vi "DataLog Subsets Actor.vi"(0 "action":T1, 5 "tag":string, 7 "subsets in":T2[](array[typedef]), 9 "tag config list":T3[](array[typedef]) {"logging parameters" format="%.2e"; "precision" items=["0", "1", "2", "3", "4", "5", "6", "7", "8", "9", "10", "11", "12", "13", "14", "15", "16", "17"]; "limit delay" format="%.2e"; "deadband" format="%.2e"}, 11 "error in (no error)":errorcluster, 12 "database path":path, 13 "new name":string) -> (4 "changes":bool, 8 "subset out":T2[](array[typedef]), 15 "error out":errorcluster)   [LabVIEW 2012]
doc: "Implements several actions designed to keep the in-memory and on-disk lists of tag subsets in sync with modifications to the tags list of their database."
uses:
  typedefs/t_Datalog Subsets Actions.ctl
  typedefs/clusters/t_DataLog Tag Subset.ctl
  typedefs/clusters/t_DataLog Tag Config.ctl
  typedefs/t_DataLog Temporal Types.ctl
  typedefs/t_DataLog Value Types.ctl
  typedefs/t_DataLog Numerical Format.ctl
  typedefs/t_DataLog Logging Algorithms.ctl
  glb_DataLog MCVD.vi
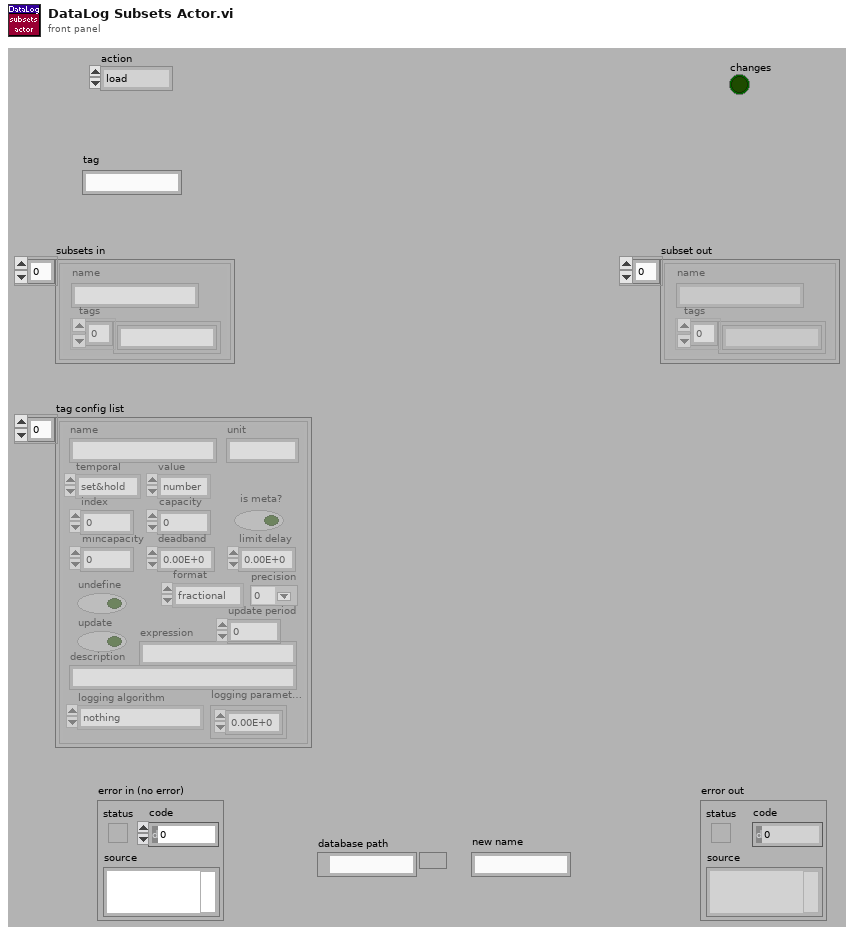
[diagram p1: front panel]
types:
  T1 = typedef "t_Datalog Subsets Actions.ctl" = enum16{"load", "rename", "delete", "save"}
  T2 = typedef "t_DataLog Tag Subset.ctl" = cluster{"name":string, "tags":string[]}
  T3 = typedef "t_DataLog Tag Config.ctl" = cluster{"name":string, "unit":string, "temporal":T4, "value":T5, "index":i32, "capacity":i32, "is meta?":bool, "mincapacity":i32, "deadband":dbl, "limit delay":dbl, "format":T6, "precision":u8, "undefine":bool, "update":bool, "update period":u16, "expression":string, "description":string, "logging algorithm":T7, "logging parameters":dbl[]}
  T4 = typedef "t_DataLog Temporal Types.ctl" = enum16{"set&hold", "sample", "event"}
  T5 = typedef "t_DataLog Value Types.ctl" = enum16{"number", "string"}
  T6 = typedef "t_DataLog Numerical Format.ctl" = enum8{"fractional", "exponential", "engineering"}
  T7 = typedef "t_DataLog Logging Algorithms.ctl" = enum16{"nothing", "changes", "everything", "every Nth", "time threshold", "value threshold + prior", "t or v threshold", "t or v threshold + prior"}
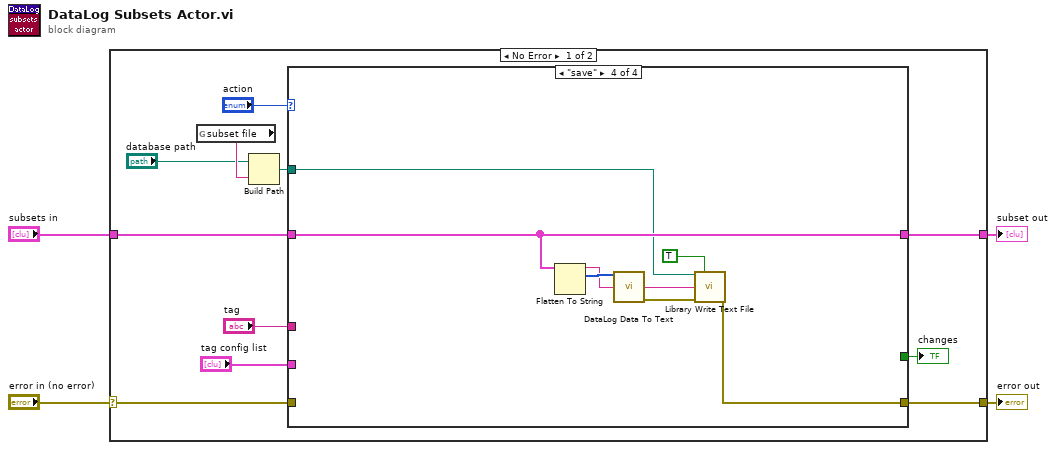
[diagram p0: block diagram]
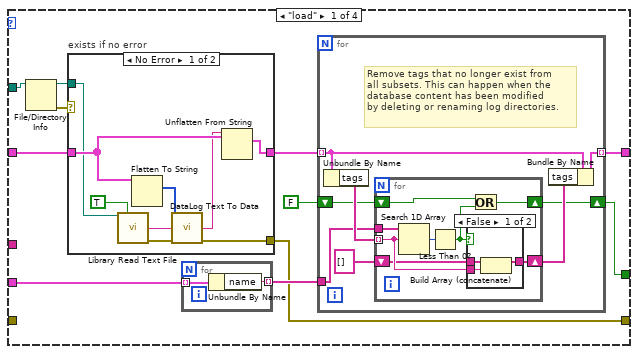
[diagram p2: hidden frame]
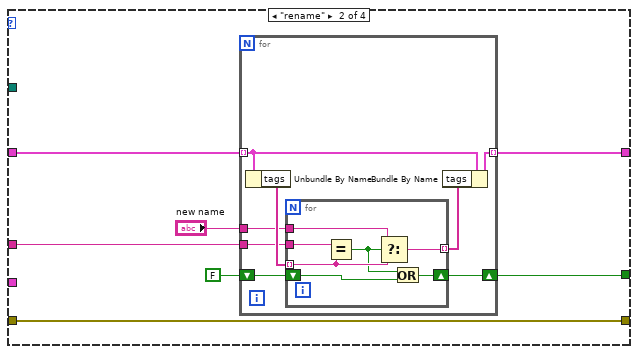
[diagram p5: hidden frame]
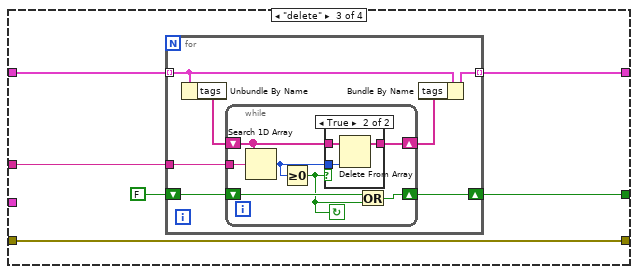
[diagram p6: hidden frame]
diagram:
  n1 = case shown="No Error" "error in (no error)" {
    selector: "error in (no error)" -> [w12 w112]
    tunnel: [w15 w113] -> w4
    tunnel: "subsets in" -> [w14 w113]
    tunnel: [w13 w112] -> w1
    frame No Error {
      n2 = global read "glb_DataLog MCVD.vi" "subset file"() -> (w8:string)
      n3 = Build Path(base path="database path", name or relative path=w8) -> (appended path=w6:path)
      n4 = case shown="\"save\"" "action" {
        tunnel: [w25 w64 w80 w105] -> w15
        tunnel: w14 -> [w23 w63 w85 w105]
        tunnel: [w20 w62 w84 w106] -> w13
        tunnel: w12 -> [_ w62 w84 _]
        tunnel: "tag" -> [_ w61 w83 _]
        tunnel: "tag config list" -> [w19 _ _ _]
        tunnel: w6 -> [w18 _ _ w104]
        tunnel: [w16 w59 w81 _] -> w5
        frame "load" {
          n5 = File/Directory Info(path=w18) -> (path out=w22:path, error out=w21:errorcluster)  [unwired: 1 in, 5 out]
          n6 = case "exists if no error" shown="No Error" w21 {
            tunnel: w23 -> [w53 _]
            tunnel: [w54 _] -> w24
            tunnel: [w51 _] -> w20
            tunnel: w22 -> [w50 _]
            frame No Error {
              n7 = call "Library Read Text File.vi"("file path"=w50, "convert eol (F)"=TRUE) -> ("read text"=w57:string, "error out"=w56:errorcluster)  [unwired: 11 in, 1 out]
              n8 = Flatten To String(anything=w53) -> (type string=w55:i16[])  [unwired: 3 in, 2 out]
              n9 = call "DataLog Text To Data.vi"("type descriptor"=w55, "text"=w57, "error in (no error)"=w56) -> ("flat data"=w52:string, "error out"=w51:errorcluster)  [unwired: 11 in]
              n10 = Unflatten From String(type=w53, binary string=w52) -> (value=w54:T2[])  [unwired: 3 in, 2 out]
            }
            frame Error {
            }
          }
          n11 = for {
            tunnel: w19 -> [w28] mode=indexing
            tunnel: [w27] -> w26 mode=indexing
            n12 = Unbundle By Name(w28) -> ("name"=w27:string)
          }
          n13 = for {
            tunnel: w24 -> [w36] mode=indexing
            tunnel: [w35] -> w25 mode=indexing
            tunnel: w26 -> [w33]
            shift-right: [w29] -> w16
            shift-left: FALSE -> [w30]
            # "Remove tags that no longer exist from\nall subsets. This can happen when the\ndatabase content has been modified\nby deleting or renaming log directories."
            n14 = Unbundle By Name(w36) -> ("tags"=w34:string[])
            n15 = for {
              tunnel: w34 -> [w42] mode=indexing
              shift-right: [w41] -> w32
              shift-left: string[] [] -> [w40]
              tunnel: w33 -> [w44]
              shift-right: [w38] -> w29
              shift-left: w30 -> [w39]
              n16 = Search 1D Array(1D array=w44, element=w42) -> (index of element=w43:i32)  [unwired: 1 in]
              n17 = Less Than 0?(x=w43) -> (x < 0?=w37:bool)
              n18 = case shown="False" w37 {
                tunnel: w42 -> [w47 _]
                tunnel: [w46 w48] -> w41
                tunnel: w40 -> [w45 w48]
                frame False {
                  n19 = Build Array (concatenate)(w45, w47) -> (w46:string[])
                }
                frame True {
                }
              }
              n20 = Or(x=w39, y=w37) -> (x .or. y?=w38:bool)
            }
            n21 = Bundle By Name(cluster=w36, "tags"=w32) -> (w35:T2)
          }
        }
        frame "rename" {
          n22 = for {
            tunnel: w63 -> [w72] mode=indexing
            tunnel: [w71] -> w64 mode=indexing
            tunnel: w61 -> [w69]
            tunnel: "new name" -> [w68]
            shift-right: [w65] -> w59
            shift-left: FALSE -> [w66]
            n23 = Unbundle By Name(w72) -> ("tags"=w70:string[])
            n24 = for {
              tunnel: w70 -> [w76] mode=indexing
              tunnel: w69 -> [w78]
              tunnel: w68 -> [w77]
              tunnel: [w79] -> w67 mode=indexing
              shift-right: [w74] -> w65
              shift-left: w66 -> [w75]
              n25 = Equal?(x=w78, y=w76) -> (x = y?=w73:bool)
              n26 = Select(t=w77, s=w73, f=w76) -> (s? t:f=w79:string)
              n27 = Or(x=w73, y=w75) -> (x .or. y?=w74:bool)
            }
            n28 = Bundle By Name(cluster=w72, "tags"=w67) -> (w71:T2)
          }
        }
        frame "delete" {
          n29 = for {
            tunnel: w85 -> [w92] mode=indexing
            tunnel: [w91] -> w80 mode=indexing
            tunnel: w83 -> [w90]
            shift-right: [w86] -> w81
            shift-left: FALSE -> [w87]
            n30 = Unbundle By Name(w92) -> ("tags"=w88:string[])
            n31 = while {
              tunnel: w90 -> [w98]
              shift-right: [w99] -> w89
              shift-left: w88 -> [w97]
              shift-right: [w93] -> w86
              shift-left: w87 -> [w95]
              stop <- w94 continue-if-true
              n32 = Search 1D Array(1D array=w97, element=w98) -> (index of element=w96:i32)  [unwired: 1 in]
              n33 = Greater Or Equal To 0?(x=w96) -> (x >= 0?=w94:bool)
              n34 = case shown="True" w94 {
                tunnel: w97 -> [w100 w103]
                tunnel: [w100 w102] -> w99
                tunnel: w96 -> [_ w101]
                frame False {
                }
                frame True {
                  n35 = Delete From Array(array=w103, index=w101) -> (array with subset deleted=w102:string[])  [unwired: 1 in, 1 out]
                }
              }
              n36 = Or(x=w95, y=w94) -> (x .or. y?=w93:bool)
            }
            n37 = Bundle By Name(cluster=w92, "tags"=w89) -> (w91:T2)
          }
        }
        frame "save" {
          n38 = Flatten To String(anything=w105) -> (data string=w109:string, type string=w111:i16[])  [unwired: 3 in, 1 out]
          n39 = call "DataLog Data To Text.vi"("type descriptor"=w111, "flat data"=w109) -> ("text"=w108:string, "error out"=w110:errorcluster)  [unwired: 12 in]
          n40 = call "Library Write Text File.vi"("file path"=w104, "convert eol (F)"=TRUE, "text to write"=w108, "error in (no error)"=w110) -> ("error out"=w106:errorcluster)  [unwired: 10 in, 1 out]
        }
      }
      "changes" <- w5
    }
    frame Error {
    }
  }
  "subset out" <- w4
  "error out" <- w1
